vi "ARC.vi"(3 "Theta_s2_init":dbl[](array[numeric]), 8 "Theta_s1_init":dbl[](array[numeric]) format="%#_f", 9 "K3":dbl[](array[numeric]), 10 "K2":dbl[](array[numeric]), 11 "K1":dbl[](array[numeric])) -> (2 "U":dbl[](array[numeric]))   [LabVIEW 2020]
uses:
  <vilib>/imath/engines/lvmath2/RunTimeEngine/Managers/WorkSpace/UID Generator.vi
  <vilib>/imath/engines/lvmath2/RunTimeEngine/IndexRead/NIMS V(S).vi
  <instcachedir>/0/NIMS V(S)_0488751826AF41519A22953C041130DC.lvgen/NIMS V(S)_0488751826AF41519A22953C041130DC_000.vi
  <vilib>/imath/engines/lvmath2/RunTimeEngine/ErrorHandling/NIMS_Create Error From Enums.vi
  <vilib>/imathl/engines/lvmath/Functions/Error Handling/Create Error.vi
  <vilib>/imath/engines/lvmath2/RunTimeEngine/RangeToken/NIMS_Range_R2 - Integer.vi
  <instcachedir>/0/NIMS_Range_R2 - Integer_FFC1A4B1B9F04947ABCB56F009996D55.lvgen/NIMS_Range_R2 - Integer_FFC1A4B1B9F04947ABCB56F009996D55_000.vi
  <vilib>/imath/engines/lvmath2/RunTimeEngine/CommandStatement/MC_CommandStatement_break.vi
  <vilib>/imath/engines/lvmath2/RunTimeEngine/IndexReplace/NIMS V(S)=S.vi
  <instcachedir>/0/NIMS V(S)=S_36728E0438CF49488BD4AB9ABCA5ECA4.lvgen/NIMS V(S)=S_36728E0438CF49488BD4AB9ABCA5ECA4_001.vi
  <vilib>/imath/engines/lvmath2/RunTimeEngine/BuiltInFunctions/diag/NIMS_diag.vi
  <instcachedir>/0/NIMS_diag_5DC8FB40F025456A81838E2C880FD792.lvgen/NIMS_diag_5DC8FB40F025456A81838E2C880FD792_002.vi
  <vilib>/imath/engines/lvmath2/RunTimeEngine/ArithmeticOperatorToken/NIMS_ArithmeticOperator_minus.vi
  <instcachedir>/0/NIMS_ArithmeticOperator_minus_822089A08BE049DB927E6BEA78E100F1.lvgen/NIMS_ArithmeticOperator_minus_822089A08BE049DB927E6BEA78E100F1_003.vi
  <vilib>/imath/engines/lvmath2/RunTimeEngine/ArithmeticOperatorToken/NIMS_ArithmeticOperator_plus.vi
  <instcachedir>/0/NIMS_ArithmeticOperator_plus_54468E2FAC2848C4BF0D457641184E60.lvgen/NIMS_ArithmeticOperator_plus_54468E2FAC2848C4BF0D457641184E60_004.vi
  <vilib>/imath/engines/lvmath2/RunTimeEngine/RunTimeType/NIMS_RunTimeType_From StrictType (excl LVString).vi
  <instcachedir>/0/NIMS_RunTimeType_From StrictType (excl LVString)_283B1B2000484AAA8744D21CE97EA49F.lvgen/NIMS_RunTimeType_From StrictType (excl LVString)_283B1B2000484AAA8744D21CE97EA49F_000.vi
  <vilib>/imath/engines/lvmath2/RunTimeEngine/LocalVariableDefStatement/MC_LocalVariableDefStatement_Display.vi
  <vilib>/imath/engines/lvmath2/RunTimeEngine/IndexRead/NIMS V(R2).vi
  <instcachedir>/0/NIMS V(R2)_C76619605A0E4E9F8B2FA9389712AC47.lvgen/NIMS V(R2)_C76619605A0E4E9F8B2FA9389712AC47_000.vi
  <vilib>/imath/engines/lvmath2/RunTimeEngine/ArithmeticOperatorToken/NIMS_ArithmeticOperator_times.vi
  <instcachedir>/0/NIMS_ArithmeticOperator_times_E1747072C05B43E9AAEA71FEEAEB18C8.lvgen/NIMS_ArithmeticOperator_times_E1747072C05B43E9AAEA71FEEAEB18C8_007.vi
  <instcachedir>/0/NIMS_ArithmeticOperator_minus_822089A08BE049DB927E6BEA78E100F1.lvgen/NIMS_ArithmeticOperator_minus_822089A08BE049DB927E6BEA78E100F1_002.vi
  <vilib>/imath/engines/lvmath2/RunTimeEngine/ArithmeticOperatorToken/NIMS_ArithmeticOperator_multmx.vi
  <instcachedir>/0/NIMS_ArithmeticOperator_multmx_177F0753FB7A49B190E35F5DD0E80316.lvgen/NIMS_ArithmeticOperator_multmx_177F0753FB7A49B190E35F5DD0E80316_004.vi
  <vilib>/imath/engines/lvmath2/RunTimeEngine/ArithmeticOperatorToken/NIMS_ArithmeticOperator_multmx(M,CV)-internal.vi
  <instcachedir>/0/NIMS_ArithmeticOperator_multmx(M,CV)-internal_19A14CC5BE0A4D31BE1E94A2E998D8C3.lvgen/NIMS_ArithmeticOperator_multmx(M,CV)-internal_19A14CC5BE0A4D31BE1E94A2E998D8C3_001.vi
  <instcachedir>/0/NIMS_ArithmeticOperator_plus_54468E2FAC2848C4BF0D457641184E60.lvgen/NIMS_ArithmeticOperator_plus_54468E2FAC2848C4BF0D457641184E60_003.vi
  <instcachedir>/0/NIMS_ArithmeticOperator_multmx_177F0753FB7A49B190E35F5DD0E80316.lvgen/NIMS_ArithmeticOperator_multmx_177F0753FB7A49B190E35F5DD0E80316_007.vi
  <instcachedir>/0/NIMS_ArithmeticOperator_plus_54468E2FAC2848C4BF0D457641184E60.lvgen/NIMS_ArithmeticOperator_plus_54468E2FAC2848C4BF0D457641184E60_011.vi
  <instcachedir>/0/NIMS_ArithmeticOperator_minus_822089A08BE049DB927E6BEA78E100F1.lvgen/NIMS_ArithmeticOperator_minus_822089A08BE049DB927E6BEA78E100F1_011.vi
  <instcachedir>/0/NIMS_ArithmeticOperator_multmx_177F0753FB7A49B190E35F5DD0E80316.lvgen/NIMS_ArithmeticOperator_multmx_177F0753FB7A49B190E35F5DD0E80316_003.vi
  <vilib>/imath/engines/lvmath2/RunTimeEngine/ArithmeticOperatorToken/NIMS_ArithmeticOperator_multmx(M,CV).vi
  <instcachedir>/0/NIMS_ArithmeticOperator_multmx(M,CV)_6A1ED936907E4DE39F29C31CF1EB9098.lvgen/NIMS_ArithmeticOperator_multmx(M,CV)_6A1ED936907E4DE39F29C31CF1EB9098_003.vi
  <instcachedir>/0/NIMS_ArithmeticOperator_minus_822089A08BE049DB927E6BEA78E100F1.lvgen/NIMS_ArithmeticOperator_minus_822089A08BE049DB927E6BEA78E100F1_008.vi
  <instcachedir>/0/NIMS_ArithmeticOperator_times_E1747072C05B43E9AAEA71FEEAEB18C8.lvgen/NIMS_ArithmeticOperator_times_E1747072C05B43E9AAEA71FEEAEB18C8_012.vi
  <instcachedir>/0/NIMS_ArithmeticOperator_plus_54468E2FAC2848C4BF0D457641184E60.lvgen/NIMS_ArithmeticOperator_plus_54468E2FAC2848C4BF0D457641184E60_002.vi
  <vilib>/imath/engines/lvmath2/RunTimeEngine/ArithmeticOperatorToken/NIMS_ArithmeticOperator_rightdiv(C,C).vi
  <instcachedir>/0/NIMS_ArithmeticOperator_rightdiv(C,C)_34A6183377BA4447889BB2F60308B12E.lvgen/NIMS_ArithmeticOperator_rightdiv(C,C)_34A6183377BA4447889BB2F60308B12E_001.vi
  <vilib>/imath/engines/lvmath2/RunTimeEngine/IndexRead/NIMS M(S).vi
  <instcachedir>/0/NIMS M(S)_B826C018497E4940AE96BD27B540B6FB.lvgen/NIMS M(S)_B826C018497E4940AE96BD27B540B6FB_004.vi
  <vilib>/imath/engines/lvmath2/RunTimeEngine/IndexReplace/NIMS M(S)=S.vi
  <instcachedir>/0/NIMS M(S)=S_033E230F5F1E47BAA81748F03F1A64B6.lvgen/NIMS M(S)=S_033E230F5F1E47BAA81748F03F1A64B6_002.vi
  <vilib>/imath/engines/lvmath2/RunTimeEngine/NodeEndStatement/NIMS_NodeEndStatement_Get Vector.vi
  <instcachedir>/0/NIMS_NodeEndStatement_Get Vector_F9EEA26507564AFBA1E30D500A99934B.lvgen/NIMS_NodeEndStatement_Get Vector_F9EEA26507564AFBA1E30D500A99934B_003.vi
  <vilib>/imath/engines/lvmath/Functions/Error Handling/MergeErrorsWrapper.vi
  <vilib>/imath/engines/lvmath2/RunTimeEngine/Managers/SymbolTable/Clear UID.vi
  <vilib>/imath/engines/lvmath2/RunTimeEngine/NodeEndStatement/NIMS_NodeEndStatement_Output.vi
  <instcachedir>/0/NIMS_NodeEndStatement_Output_53EC0D466D134D7ABD903AC30B43404B.lvgen/NIMS_NodeEndStatement_Output_53EC0D466D134D7ABD903AC30B43404B_000.vi
  <instcachedir>/0/NIMS_NodeEndStatement_Output_53EC0D466D134D7ABD903AC30B43404B.lvgen/NIMS_NodeEndStatement_Output_53EC0D466D134D7ABD903AC30B43404B_005.vi
  <vilib>/imath/engines/lvmath2/RunTimeEngine/ErrorHandling/NIMS_Finalize Error.vi
  <vilib>/imath/engines/lvmath2/RunTimeEngine/Managers/SymbolTable/NIMS_WorkSpace.lvlib
panel:
  out "A_Q":cdb[](array[numeric])
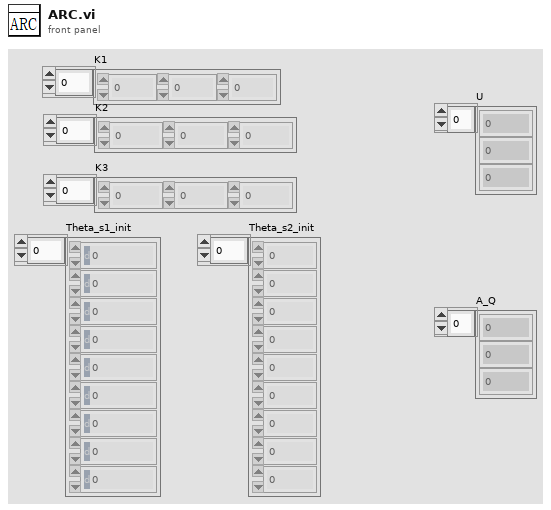
[diagram p1: front panel]
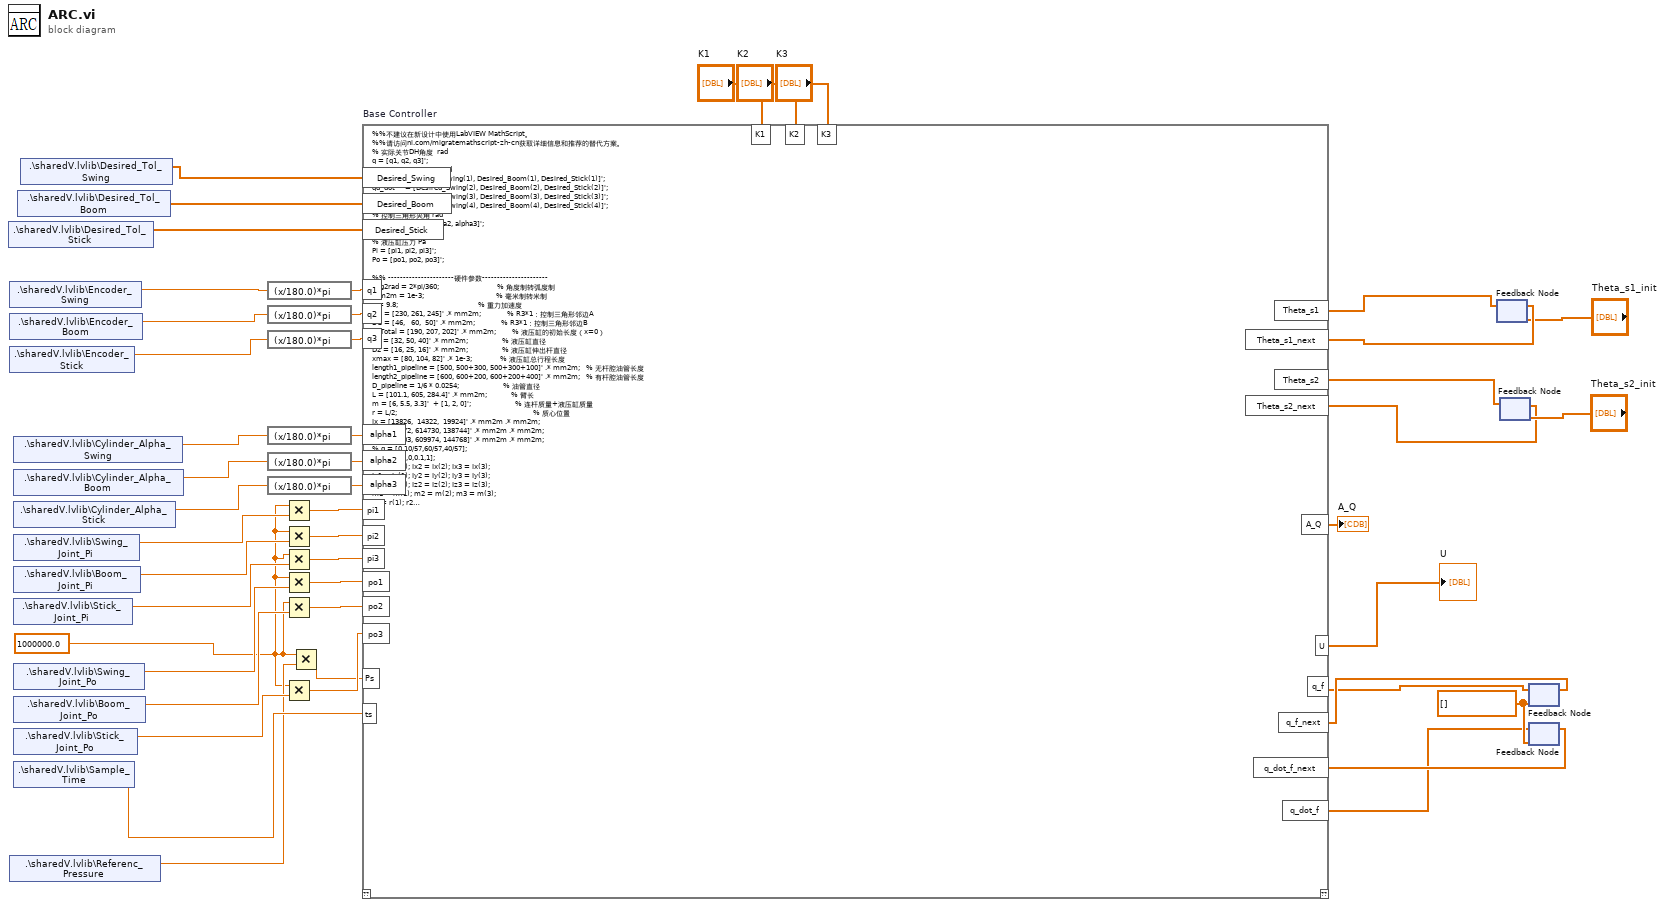
[diagram p0: block diagram]
diagram:
  w9 = 1000000.0
  w22 = dbl[] []
  n1 = shared-variable ".\\sharedV.lvlib\\Desired_Tol_Stick"() -> (w15:dbl[])  [unwired: 1 in, 1 out]
  n2 = shared-variable ".\\sharedV.lvlib\\Encoder_Swing"() -> (w47:dbl)  [unwired: 1 in, 1 out]
  n3 = shared-variable ".\\sharedV.lvlib\\Encoder_Boom"() -> (w46:dbl)  [unwired: 1 in, 1 out]
  n4 = shared-variable ".\\sharedV.lvlib\\Encoder_Stick"() -> (w45:dbl)  [unwired: 1 in, 1 out]
  n5 = shared-variable ".\\sharedV.lvlib\\Referenc_Pressure"() -> (w16:dbl)  [unwired: 1 in, 1 out]
  n6 = shared-variable ".\\sharedV.lvlib\\Cylinder_Alpha_Swing"() -> (w41:dbl)  [unwired: 1 in, 1 out]
  n7 = shared-variable ".\\sharedV.lvlib\\Cylinder_Alpha_Boom"() -> (w38:dbl)  [unwired: 1 in, 1 out]
  n8 = shared-variable ".\\sharedV.lvlib\\Cylinder_Alpha_Stick"() -> (w37:dbl)  [unwired: 1 in, 1 out]
  n9 = shared-variable ".\\sharedV.lvlib\\Swing_Joint_Pi"() -> (w35:dbl)  [unwired: 1 in, 1 out]
  n10 = shared-variable ".\\sharedV.lvlib\\Boom_Joint_Pi"() -> (w33:dbl)  [unwired: 1 in, 1 out]
  n11 = shared-variable ".\\sharedV.lvlib\\Stick_Joint_Pi"() -> (w32:dbl)  [unwired: 1 in, 1 out]
  n12 = shared-variable ".\\sharedV.lvlib\\Swing_Joint_Po"() -> (w31:dbl)  [unwired: 1 in, 1 out]
  n13 = shared-variable ".\\sharedV.lvlib\\Boom_Joint_Po"() -> (w30:dbl)  [unwired: 1 in, 1 out]
  n14 = shared-variable ".\\sharedV.lvlib\\Stick_Joint_Po"() -> (w29:dbl)  [unwired: 1 in, 1 out]
  n15 = shared-variable ".\\sharedV.lvlib\\Sample_Time"() -> (w23:dbl)  [unwired: 1 in, 1 out]
  n16 = shared-variable ".\\sharedV.lvlib\\Desired_Tol_Boom"() -> (w14:dbl[])  [unwired: 1 in, 1 out]
  n17 = shared-variable ".\\sharedV.lvlib\\Desired_Tol_Swing"() -> (w13:dbl[])  [unwired: 1 in, 1 out]
  n18 = expression code="(x/180.0)*pi"(w47) -> (w44:dbl)
  n19 = expression code="(x/180.0)*pi"(w46) -> (w43:dbl)
  n20 = expression code="(x/180.0)*pi"(w45) -> (w42:dbl)
  n21 = expression code="(x/180.0)*pi"(w41) -> (w40:dbl)
  n22 = expression code="(x/180.0)*pi"(w38) -> (w39:dbl)
  n23 = expression code="(x/180.0)*pi"(w37) -> (w36:dbl)
  n24 = Multiply(x=w9, y=w35) -> (x*y=w34:dbl)
  n25 = Multiply(x=w9, y=w33) -> (x*y=w24:dbl)
  n26 = Multiply(x=w9, y=w32) -> (x*y=w25:dbl)
  n27 = Multiply(x=w9, y=w31) -> (x*y=w26:dbl)
  n28 = Multiply(x=w9, y=w30) -> (x*y=w27:dbl)
  n29 = Multiply(x=w9, y=w29) -> (x*y=w28:dbl)
  n30 = Multiply(x=w9, y=w16) -> (x*y=w17:dbl)
  n31 = feedback #1("Theta_s1_init") -> (w7:dbl[])
  n32 = feedback #2("Theta_s2_init") -> (w3:dbl[])
  n33 = feedback #3(w22) -> (w20:dbl[])
  n34 = feedback #4(w22) -> (w18:dbl[])
  n35 = mathscript code="%%不建议在新设计中使用LabVIEW MathScript。\n%%请访问ni.com/migratemathscript-zh-cn获取详细信息和推荐的替代方案。\n% 实际关节DH角度  rad\nq = [q1, q2, q3]';\n% 期望轨迹数据重组  rad\nqd           = [Desired_Swing(1), Desired_Boom(1), Desired_Stick(1)]';\nqd_dot     = [Desired_Swing(2), Desired_Boom(2), Desired_Stick(2)]';\nqd_ddot   = [Desired_Swing(3), Desired_Boom(3), Desired_Stick(3)]';\nqd_dddot = [Desired_Swing(4), Desired_Boom(4), Desired_Stick(4)]';\n% 控制三角形夹角 rad\nalpha = [alpha1, alpha2, alpha3]'; \n\n% 液压缸压力 Pa\nPi = [pi1, pi2, pi3]';\nPo = [po1, po2, po3]';\n\n%% ----------------------硬件参数----------------------\ndeg2rad = 2*pi/360;                             % 角度制转弧度制\nmm2m = 1e-3;                                    % 毫米制转米制\ng = 9.8;                                        % 重力加速度\nAB = [230, 261, 245]' .* mm2m;             % R3*1：控制三角形邻边A\nBC = [46,   60,  50]' .* mm2m;             % R3*1：控制三角形邻边B\nx0Total = [190, 207, 202]' .* mm2m;        % 液压缸的初始长度（x=0）\nD1 = [32, 50, 40]' .* mm2m;                 % 液压缸直径\nD2 = [16, 25, 16]' .* mm2m;                 % 液压缸伸出杆直径\nxmax = [80, 104, 82]' .* 1e-3;              % 液压缸总行程长度\nlength1_pipeline = [500, 500+300, 500+300+100]' .* mm2m;   % 无杆腔油管长度\nlength2_pipeline = [600, 600+200, 600+200+400]' .* mm2m;   % 有杆腔油管长度\nD_pipeline = 1/6 * 0.0254;                      % 油管直径\nL = [101.1, 605, 284.4]' .* mm2m;            % 臂长\nm = [6, 5.5, 3.3]'  + [1, 2, 0]';                      % 连杆质量+液压缸质量\nr = L/2;                                                                    % 质心位置\nIx = [13826,  14322,  19924]' .* mm2m .* mm2m;                        \nIy = [30072, 614730, 138744]' .* mm2m .* mm2m;                       \nIz = [21003, 609974, 144768]' .* mm2m .* mm2m;                       \n% q = [0,10/57,60/57,40/57];                                                \n% qd = [0,0,0.1,1];                                                      \nIx1 = Ix(1); Ix2 = Ix(2); Ix3 = Ix(3);\nIy1 = Iy(1); Iy2 = Iy(2); Iy3 = Iy(3);\nIz1 = Iz(1); Iz2 = Iz(2); Iz3 = Iz(3);\nm1 = m(1); m2 = m(2); m3 = m(3); \nr1 = r(1); r2 = r(2); r3 = r(3); \nL1 = L(1); L2 = L(2); L3 = L(3); \nxNowTotal = zeros(3,1);\nfor ii = 1:3\n  xNowTotal(ii) = sqrt(AB(ii)^2 + BC(ii)^2 - 2*AB(ii)*BC(ii)*cos(alpha(ii)));           \t%控制三角形中关节角对应边长\nend\npxpq = AB .* BC .* sin(alpha) ./ xNowTotal;\nJ_h = diag((AB .* BC .* sin(alpha)) ./ xNowTotal);\ninv_J_h = diag(xNowTotal./ (AB .* BC .* sin(alpha)));\n% 液压相关\nA_pipeline = 0.25*pi*D_pipeline^2;        \t        % 油管面积\nAi = 0.25*pi*D1.^2;                                 % 无杆腔面积\nAo = Ai - 0.25*pi*D2.^2;                      \t    % 有杆腔面积\nVh1 = A_pipeline .* length1_pipeline;               % 无杆腔油管油液体积\nVh2 = A_pipeline.*length2_pipeline + xmax.*Ao;      % 有杆腔油管油液体积\nxL = xNowTotal - x0Total;                           % 液压缸位移\nVi = Vh1 + Ai.*xL;                                  % 无杆腔油液总体积\nVo = Vh2 - Ao.*xL;                                  % 有杆腔油液总体积\nA_Q = Ai.^2./Vi + Ao.^2./Vo;\nB_Q = Ai ./ Vi;\nC_Q = Ao ./ Vo;\n\n\n% 二阶微分滤波求q_dot q_ddot.................\nq_dot_f = q_dot_f';\nq_f = q_f';\nq_dot = q_dot_f;\nwn = 100; % 原先是100，为了减少相位滞后，应当尽可能大\nepsilon = 0.707;\nq_ddot_f = wn.^2.*q - 2.*epsilon.*wn.*q_dot_f - wn.^2.*q_f;\nq_dot_f_next = q_dot_f + q_ddot_f.*ts;\nq_f_next = q_f + q_dot_f.*ts\nq1d = q_dot(1);  q2d = q_dot(2);  q3d = q_dot(3); \nM =...\n[Ix2/2 + Ix3/2 + Iy2/2 + Iy3/2 + Iz1 - (Ix3*cos(2*q2 + 2*q3))/2 + (Iy3*cos(2*q2 + 2*q3))/2 + L1^2*m2 + L1^2*m3 + (L2^2*m3)/2 + (L3^2*m3)/2 + m1*r1^2 + (m2*r2^2)/2 - (Ix2*cos(2*q2))/2 + (Iy2*cos(2*q2))/2 + (L2^2*m3*cos(2*q2))/2 + (m2*r2^2*cos(2*q2))/2 + (L3^2*m3*cos(2*q2 + 2*q3))/2 + 2*L1*L3*m3*cos(q2 + q3) + 2*L1*L2*m3*cos(q2) + L2*L3*m3*cos(q3) + 2*L1*m2*r2*cos(q2) + L2*L3*m3*cos(2*q2 + q3),                                                            0,                                0;\n                                                                                                                                                                                                                                                                                                                                                                                                        0, m3*L2^2 + 2*m3*cos(q3)*L2*r3 + m2*r2^2 + m3*r3^2 + Iz2 + Iz3, m3*r3^2 + L2*m3*cos(q3)*r3 + Iz3;\n                                                                                                                                                                                                                                                                                                                                                                                                        0,                             m3*r3^2 + L2*m3*cos(q3)*r3 + Iz3,                    m3*r3^2 + Iz3];\n\nC =...\n[- q2d*((m3*sin(2*q2)*L2^2)/2 + m3*sin(2*q2 + q3)*L2*L3 + L1*m3*sin(q2)*L2 + (m3*sin(2*q2 + 2*q3)*L3^2)/2 + L1*m3*sin(q2 + q3)*L3 + (m2*sin(2*q2)*r2^2)/2 + L1*m2*sin(q2)*r2 - (Ix3*sin(2*q2 + 2*q3))/2 + (Iy3*sin(2*q2 + 2*q3))/2 - (Ix2*sin(2*q2))/2 + (Iy2*sin(2*q2))/2) - q3d*((Iy3*sin(2*q2 + 2*q3))/2 - (Ix3*sin(2*q2 + 2*q3))/2 + (L3^2*m3*sin(2*q2 + 2*q3))/2 + L1*L3*m3*sin(q2 + q3) + (L2*L3*m3*sin(q3))/2 + (L2*L3*m3*sin(2*q2 + q3))/2),  -q1d*((m3*sin(2*q2)*L2^2)/2 + m3*sin(2*q2 + q3)*L2*L3 + L1*m3*sin(q2)*L2 + (m3*sin(2*q2 + 2*q3)*L3^2)/2 + L1*m3*sin(q2 + q3)*L3 + (m2*sin(2*q2)*r2^2)/2 + L1*m2*sin(q2)*r2 - (Ix3*sin(2*q2 + 2*q3))/2 + (Iy3*sin(2*q2 + 2*q3))/2 - (Ix2*sin(2*q2))/2 + (Iy2*sin(2*q2))/2),  -q1d*((Iy3*sin(2*q2 + 2*q3))/2 - (Ix3*sin(2*q2 + 2*q3))/2 + (L3^2*m3*sin(2*q2 + 2*q3))/2 + L1*L3*m3*sin(q2 + q3) + (L2*L3*m3*sin(q3))/2 + (L2*L3*m3*sin(2*q2 + q3))/2);\n                                                                                                                                                                           q1d*((m3*sin(2*q2)*L2^2)/2 + m3*sin(2*q2 + q3)*L2*L3 + L1*m3*sin(q2)*L2 + (m3*sin(2*q2 + 2*q3)*L3^2)/2 + L1*m3*sin(q2 + q3)*L3 + (m2*sin(2*q2)*r2^2)/2 + L1*m2*sin(q2)*r2 - (Ix3*sin(2*q2 + 2*q3))/2 + (Iy3*sin(2*q2 + 2*q3))/2 - (Ix2*sin(2*q2))/2 + (Iy2*sin(2*q2))/2),                                                                                                                                                                                                                                                      -L2*m3*q3d*r3*sin(q3),                                                                                                                                           -L2*m3*r3*sin(q3)*(q2d + q3d);\n                                                                                                                                                                                                                                                                              q1d*((Iy3*sin(2*q2 + 2*q3))/2 - (Ix3*sin(2*q2 + 2*q3))/2 + (L3^2*m3*sin(2*q2 + 2*q3))/2 + L1*L3*m3*sin(q2 + q3) + (L2*L3*m3*sin(q3))/2 + (L2*L3*m3*sin(2*q2 + q3))/2),                                                                                                                                                                                                                                                       L2*m3*q2d*r3*sin(q3),                                                                                                                                                                       0;];\n\nG = [                                                    0;\n    g*(m2*r2*cos(q2) + m3*r3*cos(q2 + q3) + L2*m3*cos(q2));\n                                      g*m3*r3*cos(q2 + q3);] ;\n\n\n%% 预处理\ntheta_hat1 = Theta_s1(1:3);                                              % fv\ntheta_hat2 = Theta_s1(4:6);                                              % fc\ntheta_hat3 = Theta_s1(7:9);                                              % D_Fn\ntheta_hat4 = Theta_s2(1:3);                                              % D_Qin\ntheta_hat5 = Theta_s2(4:6);                                              % D_Qon\ntheta_hat6 = Theta_s2(7);                                                 % 1/beta_e\n%%\ne1 = q - qd;\ne1_dot = q_dot - qd_dot;\nqeq_dot = qd_dot - K1.*e1;\nqeq_ddot = qd_ddot - K1.*e1_dot;\ne2 = q_dot - qeq_dot;\nS_qdot = 2/pi*atan(900*q_dot);   \nFLda1 = inv_J_h * (M * qeq_dot + C*qd_dot + G);\nFLds1 = - K2 .* e2;\nFLda2 = 0;\nFLds2 = 0;\nFLd = FLda1 + FLda2 + FLds1 + FLds2;\nFL = Pi.*Ai - Po.*Ao; \ne3 = FL - FLd;\n\n% step 2\n\nFLdc_dot = ones(3,1);\n\n% QLda1 = J_h*A_Q*q_dot - B_Q*theta_hat4 - C_Q*theta_hat5 + FLdc_dot*theta_hat6 + Upsilon_Q;\nQLda1 = J_h*diag(A_Q)*qd_dot - diag(B_Q)*theta_hat4 - diag(C_Q)*theta_hat5 + FLdc_dot*theta_hat6;\nQLda2 = 0;\nQLds1 = -K3 .* e3;                                           %%%%%%%%%%%%%%%%%%%%%%%%%%%%%%%%%%%%%%%%%%%%%\nQLd = QLda1 + QLda2 +  QLds1;\n% QLd = QLds1;\n\n%% Update\nTheta_s1_next = Theta_s1;\nTheta_s2_next = Theta_s2;\n\n%%\n% Q to U\nPr = 0;                                     \nkq1 = 1.069e-9;                         \t\nkq2 = 1.069e-9;                           \t\nk = 10;                                    \t\n\nif QLd > 0 % forword\n    Delta_p1 = Ps - Pi;\n    Delta_p2 = Po - Pr;\nelse % backspacings\n    Delta_p1 = Pi - Pr;\n    Delta_p2 = Ps - Po;\nend\n\nXv = QLd ./ (Ai./Vi.*kq1.*sqrt(Delta_p1) + Ao./Vo.*kq2.*sqrt(Delta_p2));\nU = 1./k .* Xv;                            \t\n\nUmax = 5;\nfor idx = 1:3\n    if U(idx) > Umax\n        U(idx) = Umax;\n    end\n    if U(idx) < -Umax\n        U(idx) = -Umax;\n    end\nend" "Base Controller"("q1"=w44, "q2"=w43, "q3"=w42, "alpha1"=w40, "alpha2"=w39, "alpha3"=w36, "pi1"=w34, "pi2"=w24, "pi3"=w25, "po1"=w26, "po2"=w27, "po3"=w28, "ts"=w23, "q_dot_f"=w18, "q_f"=w20, "Ps"=w17, "Desired_Swing"=w13, "Desired_Boom"=w14, "Desired_Stick"=w15, "K1"="K1", "K2"="K2", "K3"="K3", "Theta_s1"=w7, "Theta_s2"=w3) -> ("q_f_next"=w21:dbl[], "q_dot_f_next"=w19:dbl[], "Theta_s2_next"=w4:dbl[], "Theta_s1_next"=w8:dbl[], "U"=→"U":dbl[], "A_Q"=→"A_Q":cdb[])  [unwired: 1 in, 1 out]
  n36 = feedback-in #1(w8) -> ()
  n37 = feedback-in #2(w4) -> ()
  n38 = feedback-in #3(w21) -> ()
  n39 = feedback-in #4(w19) -> ()
